vi "GetIPString.vi"(10 "Out_IP Address":T1 caption="Info_IP Address" {"Manual_IP"."IP4" format="%.03d"; "Manual_IP"."IP3" format="%.03d"; "Manual_IP"."IP2" format="%.03d"; "Manual_IP"."IP1" format="%.03d"; "Auto_IP"."IP3" format="%.03d"; "Auto_IP"."IP2" format="%.03d"; "Auto_IP"."IP1" format="%.03d"}) -> (1 "Net address":u32 format="%.0x")   [LabVIEW 2015]
panel:
  # "．"
  # "．"
  # "．"
  # "．"
  # "．"
  # "．"
  # "XXX"
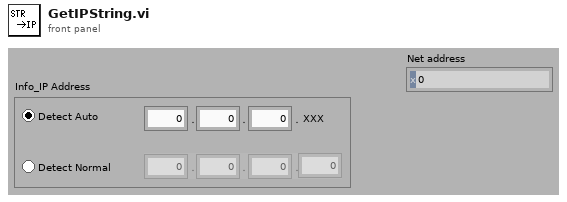
[diagram p1: front panel]
types:
  T1 = cluster{"Detect Select BOX":enum32{"Detect Auto", "Detect Normal"}, "Auto_IP":cluster{"IP1":u8, "IP2":u8, "IP3":u8}, "Manual_IP":cluster{"IP1":u8, "IP2":u8, "IP3":u8, "IP4":u8}}
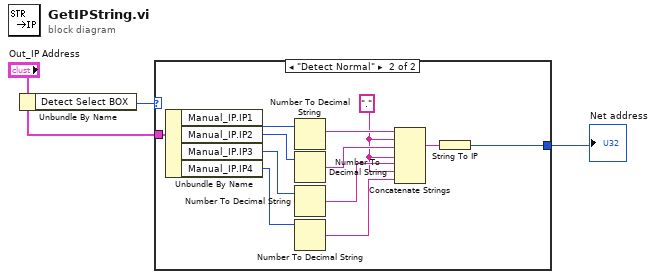
[diagram p0: block diagram]
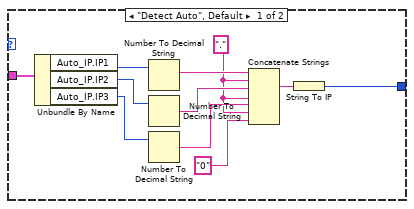
[diagram p2: hidden frame]
diagram:
  n1 = Unbundle By Name("Out_IP Address") -> ("Detect Select BOX"=w3:enum32{"Detect Auto", "Detect Normal"})
  n2 = case shown="\"Detect Normal\"" w3 {
    tunnel: "Out_IP Address" -> [w11 w23]
    tunnel: [w6 w18] -> w1
    frame "Detect Auto", Default {
      w5 = "."
      n3 = Unbundle By Name(w11) -> ("Auto_IP.IP1"=w12:u8, "Auto_IP.IP2"=w13:u8, "Auto_IP.IP3"=w14:u8)
      n4 = Number To Decimal String(number=w12) -> (decimal integer string=w10:string)  [unwired: 1 out]
      n5 = Number To Decimal String(number=w13) -> (decimal integer string=w9:string)  [unwired: 1 out]
      n6 = Number To Decimal String(number=w14) -> (decimal integer string=w8:string)  [unwired: 1 out]
      n7 = Concatenate Strings(w10, w5, w9, w5, w8, w5, "0" ("文字列")) -> (w7:string)
      n8 = String To IP(1:w7) -> (0:w6:u32)
    }
    frame "Detect Normal" {
      w17 = "."
      n9 = Unbundle By Name(w23) -> ("Manual_IP.IP1"=w24:u8, "Manual_IP.IP2"=w25:u8, "Manual_IP.IP3"=w26:u8, "Manual_IP.IP4"=w16:u8)
      n10 = Number To Decimal String(number=w24) -> (decimal integer string=w22:string)  [unwired: 1 out]
      n11 = Number To Decimal String(number=w25) -> (decimal integer string=w21:string)  [unwired: 1 out]
      n12 = Number To Decimal String(number=w26) -> (decimal integer string=w20:string)  [unwired: 1 out]
      n13 = Number To Decimal String(number=w16) -> (decimal integer string=w15:string)  [unwired: 1 out]
      n14 = Concatenate Strings(w22, w17, w21, w17, w20, w17, w15) -> (w19:string)
      n15 = String To IP(1:w19) -> (0:w18:u32)
    }
  }
  "Net address" <- w1
